vi "MultilineString_to_ArrayofStrings.vi"(0 "String 1":string, 1 "NewLineString":string="\n") -> (2 "String Array":string[](array[string]))   [LabVIEW 2011]
panel:
  # "only 1 char!"
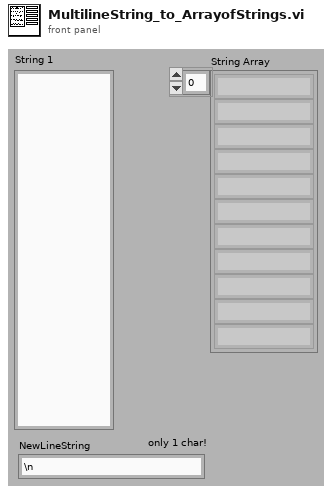
[diagram p1: front panel]
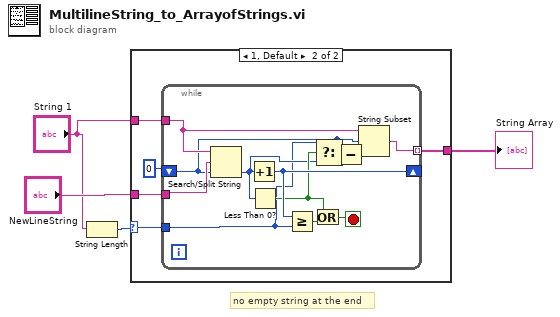
[diagram p0: block diagram]
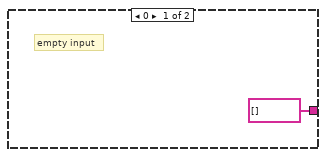
[diagram p2: hidden frame]
diagram:
  # "no empty string at the end"
  n1 = String Length(string="String 1") -> (length=w1:i32)
  n2 = case shown="1, Default" w1 {
    selector: w1 -> [_ w6]
    tunnel: [string[] [] w10] -> w4
    tunnel: "NewLineString" -> [_ w9]
    tunnel: "String 1" -> [_ w7]
    frame 0 {
      # "empty input"
    }
    frame 1, Default {
      n3 = while {
        tunnel: [w18] -> w10 mode=indexing
        tunnel: w9 -> [w22]
        shift-right: [w15] -> _
        shift-left: 0 ("offset of match") -> [w19]
        tunnel: w7 -> [w21]
        tunnel: w6 -> [w12]
        stop <- w16 stop-if-true
        n4 = Search/Split String(string=w21, search string/char (-)=w22, offset (0)=w19) -> (offset of match=w13:i32)  [unwired: 2 out]
        n5 = Increment(x=w13) -> (x+1=w15:i32)
        n6 = Less Than 0?(x=w13) -> (x < 0?=w14:bool)
        n7 = Greater Or Equal?(x=w15, y=w12) -> (x >= y?=w17:bool)
        n8 = Or(x=w14, y=w17) -> (x .or. y?=w16:bool)
        n9 = Select(t=w12, s=w14, f=w13) -> (s? t:f=w11:i32)
        n10 = Subtract(x=w11, y=w19) -> (x-y=w20:i32)
        n11 = String Subset(string=w21, offset (0)=w19, length (rest)=w20) -> (substring=w18:string)
      }
    }
  }
  "String Array" <- w4
